vi "Write Mode.vi"(8 "Error In":errorcluster, 10 "Mode":T1, 11 "Session In":refnum<class "Session.lvclass">) -> (0 "Error Out":errorcluster, 3 "Sesssion Out":refnum<class "Session.lvclass">)   [LabVIEW 2017, in "Toolkit.lvlib" / "Session.lvclass"]
uses:
  Session.lvclass
  Typedefs/Modes.ctl
  Session.lvclass/Session.ctl
  Toolkit.lvlib
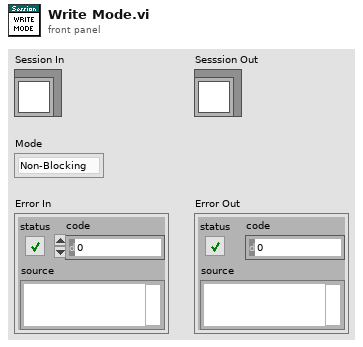
[diagram p1: front panel]
types:
  T1 = typedef "Toolkit.lvlib/Session.lvclass/Modes.ctl" = enum32{"Non-Blocking", "Blocking"}
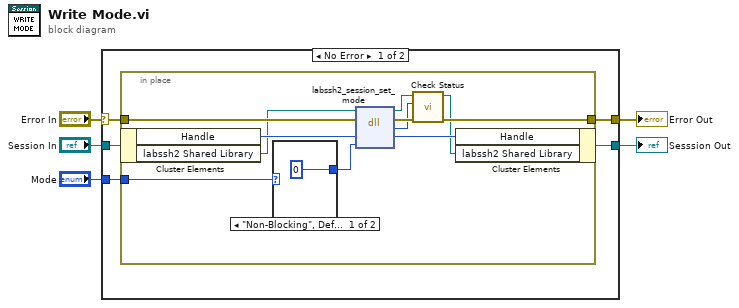
[diagram p0: block diagram]
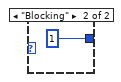
[diagram p2: hidden frame]
diagram:
  n1 = case shown="No Error" "Error In" {
    selector: "Error In" -> [w9 w25]
    tunnel: [w10 w25] -> w4
    tunnel: "Session In" -> [w8 w24]
    tunnel: [w7 w24] -> w2
    tunnel: "Mode" -> [w6 _]
    frame No Error {
      n2 = in-place {
        in-place-border: [w14] -> w10
        in-place-border: w9 -> [w21]
        in-place-border: w6 -> [w16]
        n3 = in-place-cluster #1(w8) -> ("Handle"=w20:u64, "labssh2 Shared Library"=w18:path)
        n4 = case shown="\"Non-Blocking\", Default" w16 {
          tunnel: [0 1] -> w15
          frame "Non-Blocking", Default {
          }
          frame "Blocking" {
          }
        }
        n5 = dll-call lib="D:/Users/cfield/Code/Field R&D Services/SSH/LabSSH2/LabVIEW/trunk/src/LabSSH2/Private/labssh2.*" fn="labssh2_session_set_mode"(path in=w18, error in=w21, "session"=w20, "blocking"=w15) -> (path out=w12:path, error out=w17:errorcluster, "status"=w13:i32, "session"=w19:u64)  [unwired: 2 in]
        n6 = call "Check Status.vi"("Error In"=w17, "Status"=w13, "labssh2 Shared Library In"=w12) -> ("Error Out"=w14:errorcluster, "labssh2 Shared Library Out"=w11:path)  [unwired: 7 in]
        n7 = in-place-cluster #1("Handle"=w19, "labssh2 Shared Library"=w11) -> (w7:refnum<class "Session.lvclass">)
      }
    }
    frame Error {
    }
  }
  "Sesssion Out" <- w2
  "Error Out" <- w4
